vi "Rotate.vi"(0 "reference in":refnum<class "Gasoline Motor.lvclass">, 5 "Degree":string, 11 "Error In":errorcluster) -> (4 "reference out":refnum<class "Gasoline Motor.lvclass">, 6 "Result":string, 15 "Error Out":errorcluster)   [LabVIEW 2024, in "Gasoline Motor.lvclass"]
doc: "Turn motors rotor for given degrees"
uses:
  Gasoline Motor.lvclass
  Gasoline Motor.lvclass/Gasoline Motor.ctl
panel:
  # "Connector Pane"
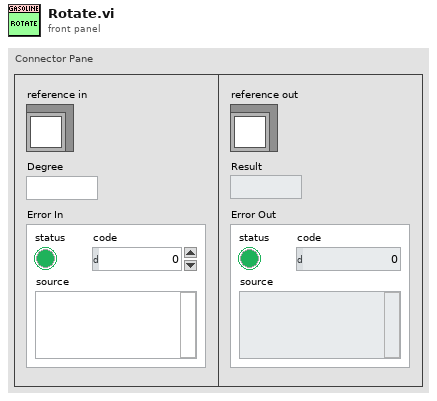
[diagram p1: front panel]
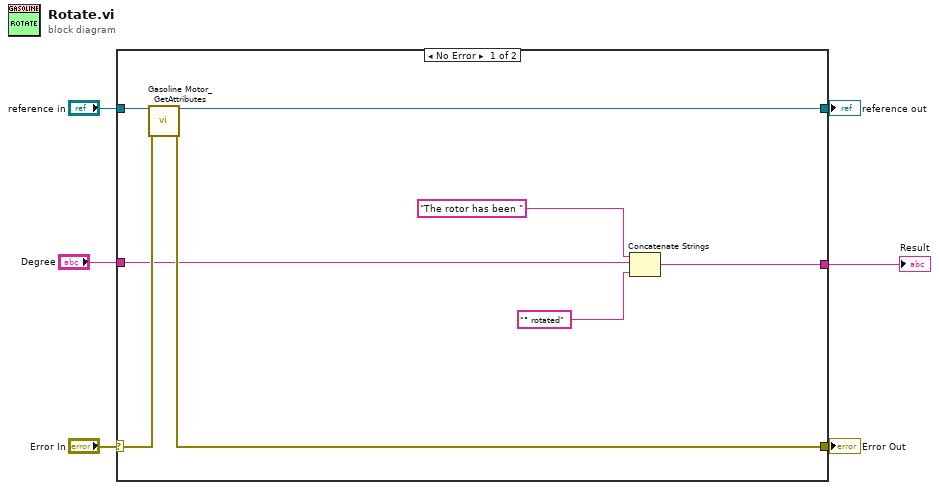
[diagram p0: block diagram]
diagram:
  n1 = case shown="No Error" "Error In" {
    selector: "Error In" -> [w14 w17]
    tunnel: [w13 w17] -> w5
    tunnel: [w11 w16] -> w3
    tunnel: "reference in" -> [w12 w16]
    tunnel: "Degree" -> [w10 w15]
    tunnel: [w7 w15] -> w1
    frame No Error {
      n2 = call "Gasoline Motor_GetAttributes.vi"("reference in"=w12, "Error In"=w14) -> ("reference out"=w11:refnum<class "Gasoline Motor.lvclass">, "Error Out"=w13:errorcluster)  [unwired: 10 in, 2 out]
      n3 = Concatenate Strings("The rotor has been " ("string"), w10, "° rotated" ("string")) -> (w7:string)
    }
    frame Error {
    }
  }
  "Error Out" <- w5
  "reference out" <- w3
  "Result" <- w1
